vi "RPN_Kalkulator.vi"() -> ()   [LabVIEW 2021]
uses:
  sm_data.ctl
panel:
  in  "Inwersja":bool
  in  "Kwadrat":bool
  in  "Negacja":bool
  in  "Pierwiastek":bool
  in  "C":bool
  in  "Enter":bool
  in  "X":dbl=95.0
  out "Z":dbl
  out "Y":dbl
  in  "Coma":bool
  in  "Dzielenie":bool
  in  "Mnożenie":bool
  in  "Odejmowanie":bool
  in  "Dodawanie":bool
  in  "0":bool
  in  "9":bool
  in  "8":bool
  in  "7":bool
  in  "6":bool
  in  "5":bool
  in  "4":bool
  in  "3":bool
  in  "2":bool
  in  "1":bool
  # "RPN\nEnter \nWprowadza dane na stos"
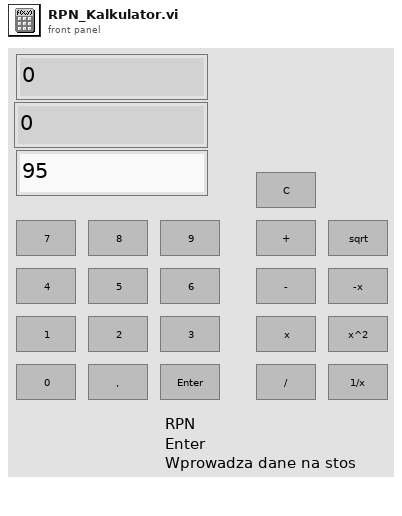
[diagram p1: front panel]
types:
  T1 = typedef "sm_data.ctl" = cluster{"number_str":string}
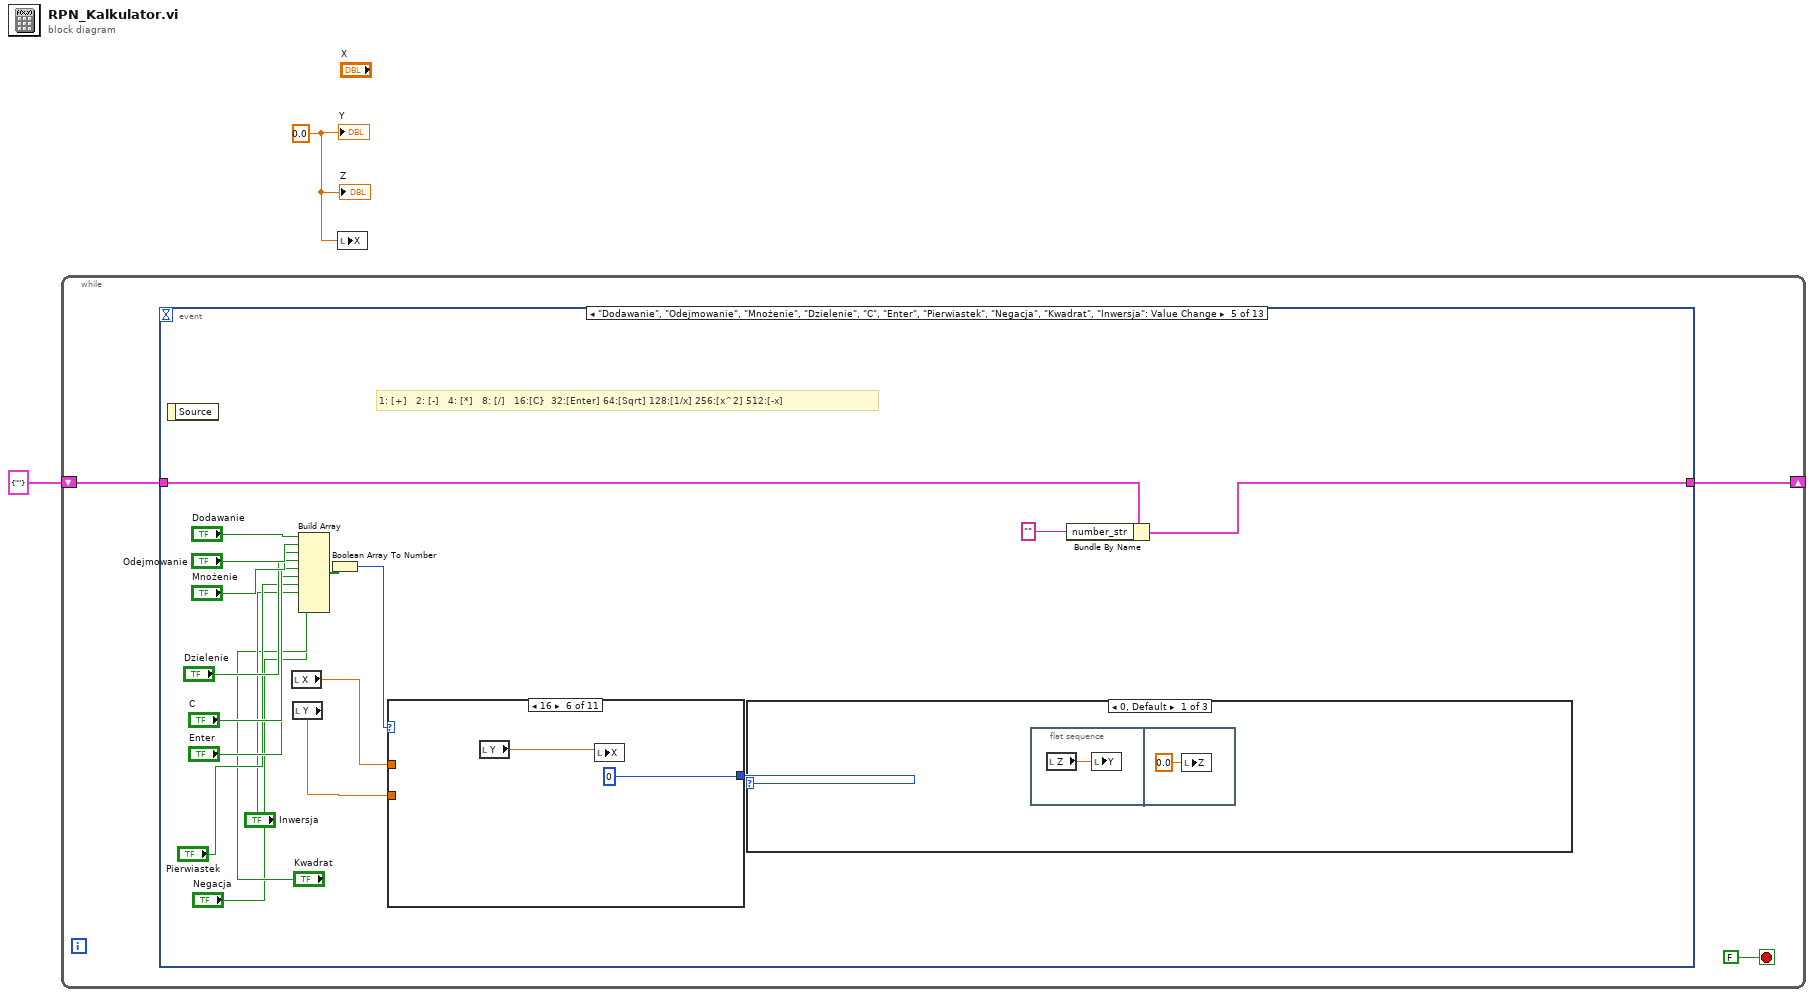
[diagram p0: block diagram]
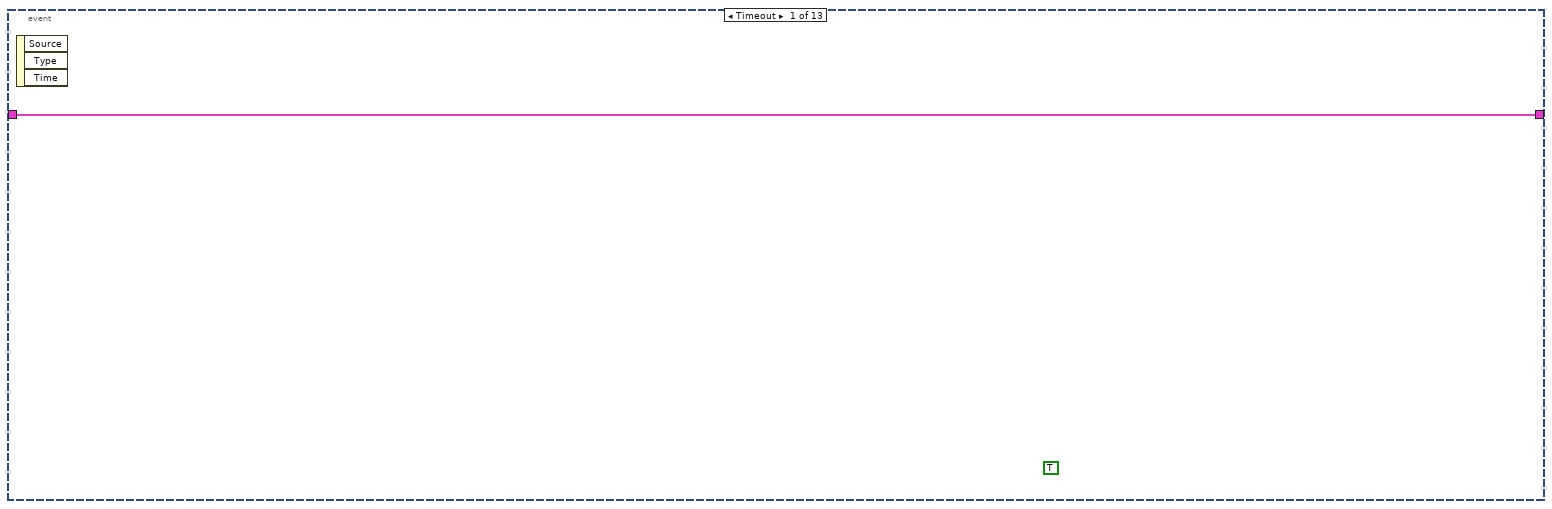
[diagram p2: hidden frame]
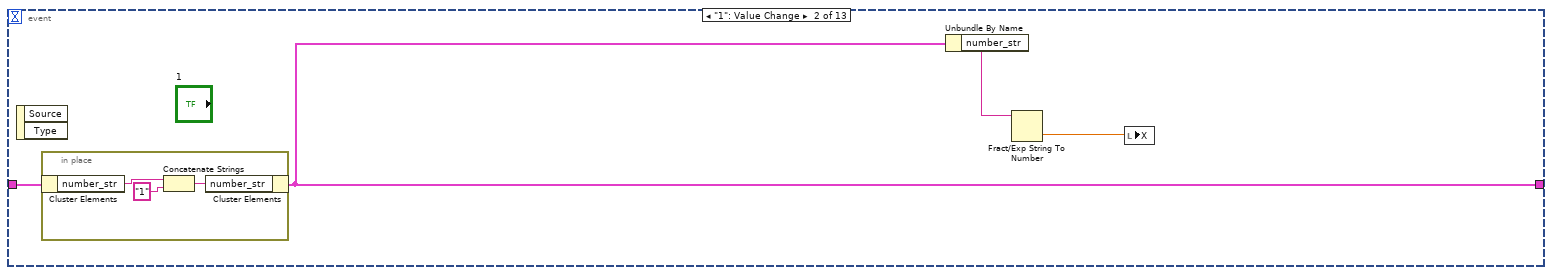
[diagram p3: hidden frame]
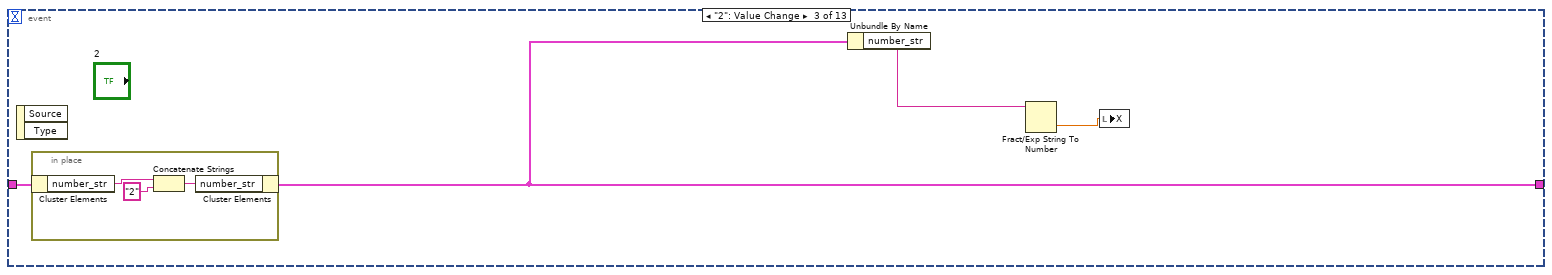
[diagram p4: hidden frame]
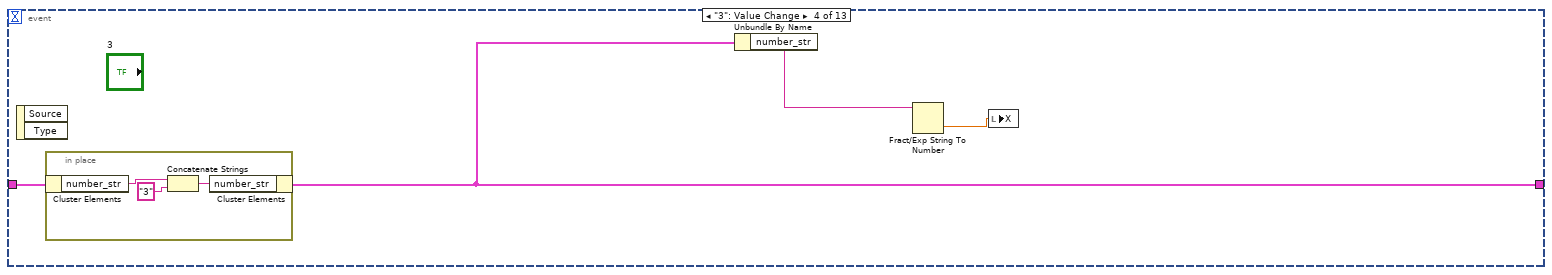
[diagram p5: hidden frame]
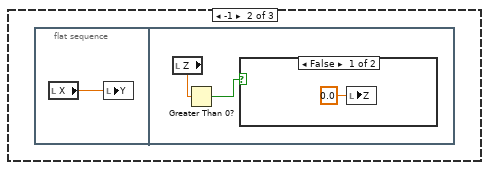
[diagram p6: hidden frame]
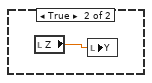
[diagram p7: hidden frame]
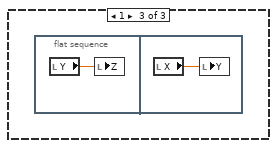
[diagram p8: hidden frame]
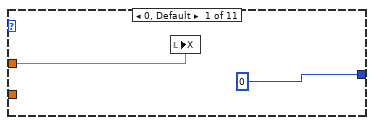
[diagram p9: hidden frame]
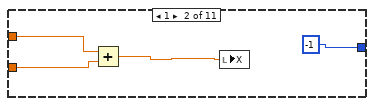
[diagram p10: hidden frame]
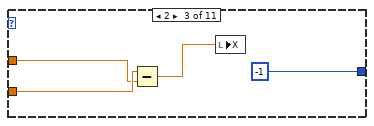
[diagram p11: hidden frame]
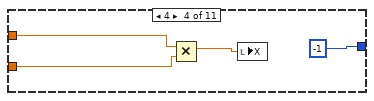
[diagram p12: hidden frame]
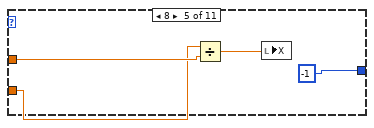
[diagram p13: hidden frame]
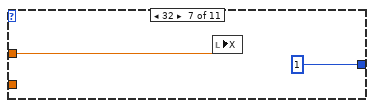
[diagram p14: hidden frame]
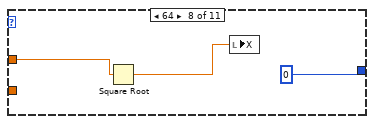
[diagram p15: hidden frame]
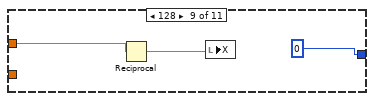
[diagram p16: hidden frame]
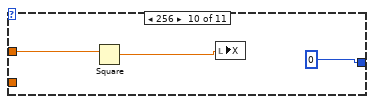
[diagram p17: hidden frame]
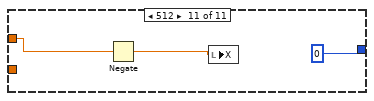
[diagram p18: hidden frame]
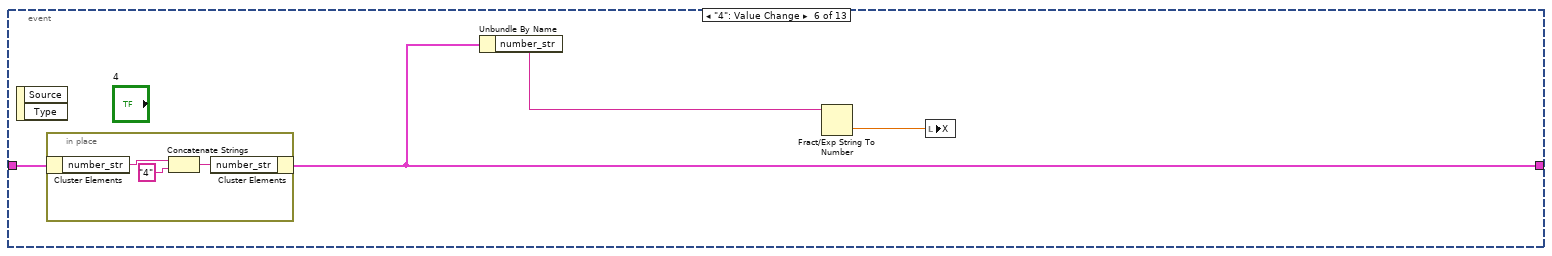
[diagram p19: hidden frame]
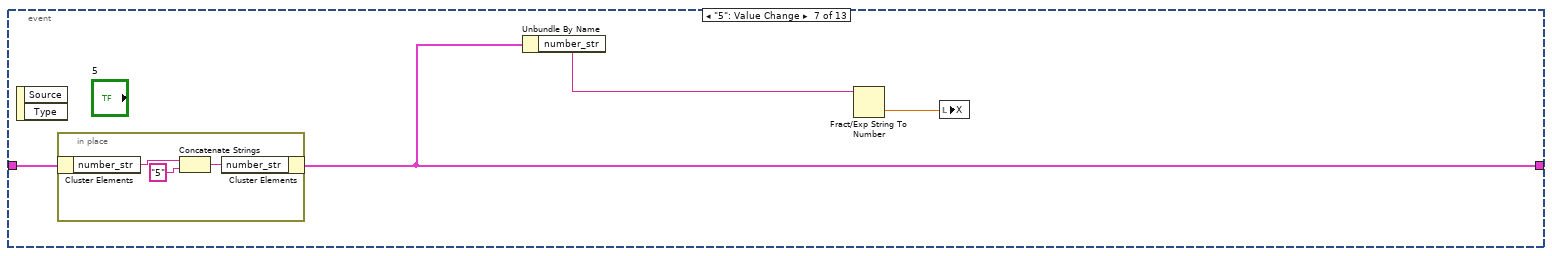
[diagram p20: hidden frame]
diagram:
  w1 = 0.0 ("Y")
  n1 = while {
    shift-right: [w4] -> _
    shift-left: T1 {"number_str"=""} -> [w5]
    stop <- FALSE stop-if-true
    n2 = event shown="[4] \"Dodawanie\", \"Odejmowanie\", \"Mnożenie\", \"Dzielenie\", \"C\", \"Enter\", \"Pierwiastek\", \"Negacja\", \"Kwadrat\", \"Inwersja\": Value Change" {
      selector: _ -> [_ _ _ _ _ _ _ _ _ _ _ _ _]
      dyn-events: _ -> [_ _ _ _ _ _ _ _ _ _ _ _ _]
      timeout: _ -> [_ _ _ _ _ _ _ _ _ _ _ _ _]
      tunnel: w5 -> [w6 w10 w17 w24 w30 w92 w99 w106 w113 w120 w127 w134 w141]
      tunnel: [w6 w9 w16 w22 w28 w90 w97 w104 w111 w118 w125 w132 w139] -> w4
      event Timeout {
        (unwired) TRUE
        n3 = event-data() -> ()  [unwired: 1 in, 3 out]
      }
      event "1": Value Change {
        n4 = event-data() -> ()  [unwired: 1 in, 2 out]
        n5 = in-place {
          n6 = in-place-cluster #1(w10) -> ("number_str"=w13:string)
          n7 = Concatenate Strings(w13, "1" ("string")) -> (w12:string)
          n8 = in-place-cluster #1("number_str"=w12) -> (w9:T1)
        }
        n9 = Unbundle By Name(w9) -> ("number_str"=w7:string)
        n10 = Fract/Exp String To Number(string=w7) -> (number=w8:dbl)  [unwired: 3 in, 1 out]
        n11 = local write "X"(w8) -> ()
      }
      event "2": Value Change {
        n12 = event-data() -> ()  [unwired: 1 in, 2 out]
        n13 = in-place {
          n14 = in-place-cluster #2(w17) -> ("number_str"=w20:string)
          n15 = Concatenate Strings(w20, "2" ("string")) -> (w19:string)
          n16 = in-place-cluster #2("number_str"=w19) -> (w16:T1)
        }
        n17 = Unbundle By Name(w16) -> ("number_str"=w15:string)
        n18 = Fract/Exp String To Number(string=w15) -> (number=w14:dbl)  [unwired: 3 in, 1 out]
        n19 = local write "X"(w14) -> ()
      }
      event "3": Value Change {
        n20 = event-data() -> ()  [unwired: 1 in, 2 out]
        n21 = in-place {
          n22 = in-place-cluster #3(w24) -> ("number_str"=w27:string)
          n23 = Concatenate Strings(w27, "3" ("string")) -> (w26:string)
          n24 = in-place-cluster #3("number_str"=w26) -> (w22:T1)
        }
        n25 = Unbundle By Name(w22) -> ("number_str"=w23:string)
        n26 = Fract/Exp String To Number(string=w23) -> (number=w21:dbl)  [unwired: 3 in, 1 out]
        n27 = local write "X"(w21) -> ()
      }
      event "Dodawanie", "Odejmowanie", "Mnożenie", "Dzielenie", "C", "Enter", "Pierwiastek", "Negacja", "Kwadrat", "Inwersja": Value Change {
        # "1: [+]   2: [-]   4: [*]   8: [/]   16:[C}  32:[Enter] 64:[Sqrt] 128:[1/x] 256:[x^2] 512:[-x]"
        n28 = event-data() -> ()  [unwired: 1 in, 1 out]
        n29 = local read "X"() -> (w39:dbl)
        n30 = local read "Y"() -> (w40:dbl)
        n31 = Build Array("Dodawanie", "Odejmowanie", "Mnożenie", "Dzielenie", "C", "Enter", "Pierwiastek", "Inwersja", "Kwadrat", "Negacja") -> (w45:bool[])
        n32 = Boolean Array To Number(Boolean array=w45) -> (number=w38:u32)
        n33 = case shown="16" w38 {
          tunnel: w40 -> [_ w60 w64 w66 w70 _ _ _ _ _ _]
          tunnel: w39 -> [w55 w59 w63 w68 w71 _ w75 w78 w81 w84 w87]
          tunnel: [0 -1 -1 -1 -1 0 1 0 0 0 0] -> w31
          frame 0, Default {
            n34 = local write "X"(w55) -> ()
          }
          frame 1 {
            n35 = Add(x=w59, y=w60) -> (x+y=w57:dbl)
            n36 = local write "X"(w57) -> ()
          }
          frame 2 {
            n37 = Subtract(x=w64, y=w63) -> (x-y=w61:dbl)
            n38 = local write "X"(w61) -> ()
          }
          frame 4 {
            n39 = Multiply(x=w68, y=w66) -> (x*y=w65:dbl)
            n40 = local write "X"(w65) -> ()
          }
          frame 8 {
            n41 = Divide(x=w70, y=w71) -> (x/y=w69:dbl)
            n42 = local write "X"(w69) -> ()
          }
          frame 16 {
            n43 = local read "Y"() -> (w73:dbl)
            n44 = local write "X"(w73) -> ()
          }
          frame 32 {
            n45 = local write "X"(w75) -> ()
          }
          frame 64 {
            n46 = Square Root(x=w78) -> (sqrt(x)=w77:dbl)
            n47 = local write "X"(w77) -> ()
          }
          frame 128 {
            n48 = Reciprocal(x=w81) -> (1/x=w80:dbl)
            n49 = local write "X"(w80) -> ()
          }
          frame 256 {
            n50 = Square(x=w84) -> (x^2=w83:dbl)
            n51 = local write "X"(w83) -> ()
          }
          frame 512 {
            n52 = Negate(x=w87) -> (-x=w86:dbl)
            n53 = local write "X"(w86) -> ()
          }
        }
        n54 = case shown="0, Default" w31 {
          frame 0, Default {
            n55 = flat-sequence {
              frame #0 {
                n56 = local read "Z"() -> (w46:dbl)
                n57 = local write "Y"(w46) -> ()
              }
              frame #1 {
                n58 = local write "Z"(0.0 ("Y")) -> ()
              }
            }
          }
          frame -1 {
            n59 = flat-sequence {
              frame #0 {
                n60 = local read "X"() -> (w48:dbl)
                n61 = local write "Y"(w48) -> ()
              }
              frame #1 {
                n62 = local read "Z"() -> (w49:dbl)
                n63 = Greater Than 0?(x=w49) -> (x > 0?=w50:bool)
                n64 = case shown="False" w50 {
                  frame False {
                    n65 = local write "Z"(0.0 ("Z")) -> ()
                  }
                  frame True {
                    n66 = local read "Z"() -> (w52:dbl)
                    n67 = local write "Y"(w52) -> ()
                  }
                }
              }
            }
          }
          frame 1 {
            n68 = flat-sequence {
              frame #0 {
                n69 = local read "Y"() -> (w53:dbl)
                n70 = local write "Z"(w53) -> ()
              }
              frame #1 {
                n71 = local read "X"() -> (w54:dbl)
                n72 = local write "Y"(w54) -> ()
              }
            }
          }
        }
        n73 = Bundle By Name(cluster=w30, "number_str"="") -> (w28:T1)
      }
      event "4": Value Change {
        n74 = event-data() -> ()  [unwired: 1 in, 2 out]
        n75 = in-place {
          n76 = in-place-cluster #4(w92) -> ("number_str"=w95:string)
          n77 = Concatenate Strings(w95, "4" ("string")) -> (w94:string)
          n78 = in-place-cluster #4("number_str"=w94) -> (w90:T1)
        }
        n79 = Unbundle By Name(w90) -> ("number_str"=w91:string)
        n80 = Fract/Exp String To Number(string=w91) -> (number=w89:dbl)  [unwired: 3 in, 1 out]
        n81 = local write "X"(w89) -> ()
      }
      event "5": Value Change {
        n82 = event-data() -> ()  [unwired: 1 in, 2 out]
        n83 = in-place {
          n84 = in-place-cluster #5(w99) -> ("number_str"=w102:string)
          n85 = Concatenate Strings(w102, "5" ("string")) -> (w101:string)
          n86 = in-place-cluster #5("number_str"=w101) -> (w97:T1)
        }
        n87 = Unbundle By Name(w97) -> ("number_str"=w98:string)
        n88 = Fract/Exp String To Number(string=w98) -> (number=w96:dbl)  [unwired: 3 in, 1 out]
        n89 = local write "X"(w96) -> ()
      }
      event "6": Value Change {
        n90 = event-data() -> ()  [unwired: 1 in, 1 out]
        n91 = in-place {
          n92 = in-place-cluster #6(w106) -> ("number_str"=w109:string)
          n93 = Concatenate Strings(w109, "6" ("string")) -> (w108:string)
          n94 = in-place-cluster #6("number_str"=w108) -> (w104:T1)
        }
        n95 = Unbundle By Name(w104) -> ("number_str"=w105:string)
        n96 = Fract/Exp String To Number(string=w105) -> (number=w103:dbl)  [unwired: 3 in, 1 out]
        n97 = local write "X"(w103) -> ()
      }
      event "7": Value Change {
        n98 = event-data() -> ()  [unwired: 1 in, 2 out]
        n99 = in-place {
          n100 = in-place-cluster #7(w113) -> ("number_str"=w116:string)
          n101 = Concatenate Strings(w116, "7" ("string")) -> (w115:string)
          n102 = in-place-cluster #7("number_str"=w115) -> (w111:T1)
        }
        n103 = Unbundle By Name(w111) -> ("number_str"=w112:string)
        n104 = Fract/Exp String To Number(string=w112) -> (number=w110:dbl)  [unwired: 3 in, 1 out]
        n105 = local write "X"(w110) -> ()
      }
      event "8": Value Change {
        n106 = event-data() -> ()  [unwired: 1 in, 2 out]
        n107 = in-place {
          n108 = in-place-cluster #8(w120) -> ("number_str"=w123:string)
          n109 = Concatenate Strings(w123, "8" ("string")) -> (w122:string)
          n110 = in-place-cluster #8("number_str"=w122) -> (w118:T1)
        }
        n111 = Unbundle By Name(w118) -> ("number_str"=w119:string)
        n112 = Fract/Exp String To Number(string=w119) -> (number=w117:dbl)  [unwired: 3 in, 1 out]
        n113 = local write "X"(w117) -> ()
      }
      event "9": Value Change {
        n114 = event-data() -> ()  [unwired: 1 in, 1 out]
        n115 = in-place {
          n116 = in-place-cluster #9(w127) -> ("number_str"=w130:string)
          n117 = Concatenate Strings(w130, "9" ("string")) -> (w129:string)
          n118 = in-place-cluster #9("number_str"=w129) -> (w125:T1)
        }
        n119 = Unbundle By Name(w125) -> ("number_str"=w126:string)
        n120 = Fract/Exp String To Number(string=w126) -> (number=w124:dbl)  [unwired: 3 in, 1 out]
        n121 = local write "X"(w124) -> ()
      }
      event "0": Value Change {
        n122 = event-data() -> ()  [unwired: 1 in, 1 out]
        n123 = in-place {
          n124 = in-place-cluster #10(w134) -> ("number_str"=w137:string)
          n125 = Concatenate Strings(w137, "0" ("string")) -> (w136:string)
          n126 = in-place-cluster #10("number_str"=w136) -> (w132:T1)
        }
        n127 = Unbundle By Name(w132) -> ("number_str"=w133:string)
        n128 = Fract/Exp String To Number(string=w133) -> (number=w131:dbl)  [unwired: 3 in, 1 out]
        n129 = local write "X"(w131) -> ()
      }
      event "Coma": Value Change {
        n130 = event-data() -> ()  [unwired: 1 in, 1 out]
        n131 = in-place {
          n132 = in-place-cluster #11(w141) -> ("number_str"=w144:string)
          n133 = Concatenate Strings(w144, "," ("string")) -> (w143:string)
          n134 = in-place-cluster #11("number_str"=w143) -> (w139:T1)
        }
        n135 = Unbundle By Name(w139) -> ("number_str"=w140:string)
        n136 = Fract/Exp String To Number(string=w140) -> (number=w138:dbl)  [unwired: 3 in, 1 out]
        n137 = local write "X"(w138) -> ()
      }
    }
  }
  n138 = local write "X"(w1) -> ()
  "Y" <- w1
  "Z" <- w1
